vi "Initialize.vi"(8 "error in":errorcluster, 11 "Plugin in":refnum<class "Test Sequencer.lvclass">) -> (0 "error out":errorcluster, 3 "Plugin out":refnum<class "Test Sequencer.lvclass">)   [LabVIEW 2020, in "Test Sequencer.lvlib" / "Test Sequencer.lvclass"]
uses:
  Test Sequencer.lvclass
  C:/Program Files/National Instruments/LabVIEW 2020/vi.lib/FlexLogger/SDK/PluginSDK.lvlibp/PEFClasses/SDK/Plugin/Plugin.lvclass
  <vilib>/FlexLogger/SDK/PluginSDK.lvlibp/PEFClasses/SDK/Processing Element/Timing Parameters.ctl
  <vilib>/FlexLogger/SDK/PluginSDK.lvlibp/PEFClasses/SDK/Processing Element/Timing Method.ctl
  Params.ctl
  Test Sequencer.lvclass/Test Sequencer.ctl
  <vilib>/FlexLogger/SDK/PluginSDK.lvlibp/PEFClasses/SDK/Producer Channel/Producer Channel.lvclass
  C:/Program Files/National Instruments/LabVIEW 2020/vi.lib/FlexLogger/SDK/PluginSDK.lvlibp/PEFClasses/SDK/Channel/Channel.lvclass
  <vilib>/FlexLogger/SDK/PluginSDK.lvlibp/PEFClasses/SDK/Plugin/ParameterAccess/Write Boolean.vi
  <vilib>/FlexLogger/SDK/PluginSDK.lvlibp/PEFClasses/SDK/Plugin/ParameterAccess/Write I32.vi
  <vilib>/FlexLogger/SDK/PluginSDK.lvlibp/PEFClasses/SDK/Plugin/ParameterAccess/Write DBL.vi
  <vilib>/FlexLogger/SDK/PluginSDK.lvlibp/PEFClasses/SDK/Producer Channel/Create Producer Channel.vi
  <vilib>/FlexLogger/SDK/PluginSDK.lvlibp/PEFClasses/SDK/Plugin/Plugin.lvclass
  <vilib>/FlexLogger/SDK/PluginSDK.lvlibp/PEFClasses/SDK/Processing Element/Processing Element.lvclass
  C:/Program Files/National Instruments/LabVIEW 2020/vi.lib/FlexLogger/SDK/PluginSDK.lvlibp/PEFClasses/SDK/Processing Element/Processing Element.lvclass
  \\nirvana\temp/bbuchanan/2020/Test Sequencer.lvclass
  <vilib>/FlexLogger/SDK/PluginSDK.lvlibp
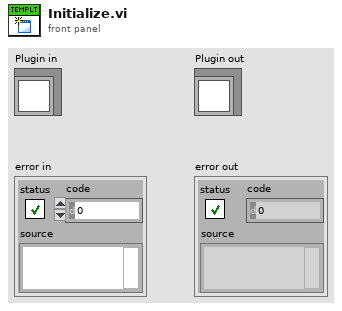
[diagram p1: front panel]
types:
  T1 = typedef "Test Sequencer.lvlib/Test Sequencer.lvclass/Params.ctl" = cluster{"Sequence Durations":dbl[], "Reset on Test Start":bool, "Current Sequence ID":u32, "Total Iterations":u32, "Last Timestamp":timestamp, "Number of Sequence Steps":i32}
  T2 = typedef "PluginSDK.lvlibp/Processing Element.lvclass/Timing Parameters.ctl" = cluster{"Timing Method":T3, "Timing Period (ms)":i32}
  T3 = typedef "PluginSDK.lvlibp/Processing Element.lvclass/Timing Method.ctl" = enum16{"Periodic", "Immediate", "On Data Ready", "Triggered"}
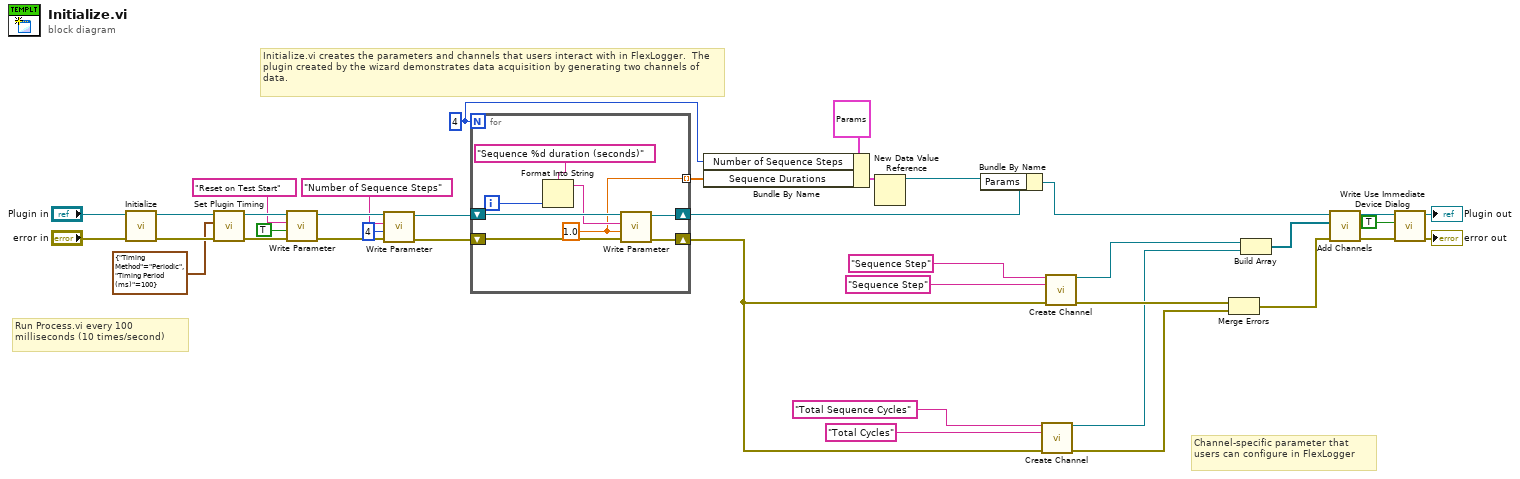
[diagram p0: block diagram]
diagram:
  w15 = 4
  # "Channel-specific parameter that users can configure in FlexLogger"
  # "Run Process.vi every 100 milliseconds (10 times/second)"
  # "Initialize.vi creates the parameters and channels that users interact with in FlexLogger.  The plugin created by the wizard demonstrates data acquisition by generating two channels of data."
  n1 = call-parent "Initialize.vi"("error in (no error)"="error in", "Plugin in"="Plugin in") -> ("error out"=w36:errorcluster, "Plugin out"=w34:refnum<class "Test Sequencer.lvclass">)  [unwired: 8 in]
  n2 = call <vilib>:"Set Plugin Timing.vi"("error in (no error)"=w36, "Timing Parameters"=T2 {"Timing Method"=enum."Periodic", "Timing Period (ms)"=100}, "Plugin in"=w34) -> ("error out"=w30:errorcluster, "Plugin out"=w31:refnum<class "Test Sequencer.lvclass">)  [unwired: 7 in]
  n3 = call-poly <vilib>:"Write Parameter.vi"("error in (no error)"=w30, "Value"=TRUE, "Name"="Reset on Test Start", "Plugin in"=w31) -> ("error out"=w21:errorcluster, "Plugin out"=w20:refnum<class "Test Sequencer.lvclass">)  [unwired: 6 in]
  n4 = call-poly <vilib>:"Write Parameter.vi"("error in (no error)"=w21, "Value"=4, "Name"="Number of Sequence Steps", "Plugin in"=w20) -> ("error out"=w16:errorcluster, "Plugin out"=w17:refnum<class "Test Sequencer.lvclass">)  [unwired: 6 in]
  n5 = for {
    N: w15 -> [_]
    shift-right: [w42] -> w27
    shift-left: w17 -> [w46]
    shift-right: [w41] -> w3
    shift-left: w16 -> [w45]
    tunnel: [w40] -> w25 mode=indexing
    i -> [w39]
    w40 = 1.0 ("Value")
    n6 = Format Into String(format string="Sequence %d duration (seconds)" ("Name"), w39) -> (resulting string=w43:string)  [unwired: 2 in, 1 out]
    n7 = call-poly <vilib>:"Write Parameter.vi"("error in (no error)"=w45, "Value"=w40, "Name"=w43, "Plugin in"=w46) -> ("error out"=w41:errorcluster, "Plugin out"=w42:refnum<class "Test Sequencer.lvclass">)  [unwired: 6 in]
  }
  n8 = Bundle By Name(cluster=T1 {"Sequence Durations"=[], "Reset on Test Start"=TRUE, "Current Sequence ID"=0, "Total Iterations"=0, "Last Timestamp"=timestamp(0 s since 1904-01-01), "Number of Sequence Steps"=0}, "Number of Sequence Steps"=w15, "Sequence Durations"=w25) -> (w24:T1)
  n9 = New Data Value Reference(data value=w24) -> (data value reference=w22:refnum<data-value>)  [unwired: 1 in, 1 out]
  n10 = Bundle By Name(cluster=w27, "Params"=w22) -> (w23:refnum<class "Test Sequencer.lvclass">)
  n11 = call-poly <vilib>:"Create Channel.vi"("Unique Channel Identifier"="Total Sequence Cycles" ("format string"), "Default Channel Name"="Total Cycles" ("format string"), "error in (no error)"=w3) -> ("Producer Channel"=w1:refnum<class "Producer Channel.lvclass">, "error out"=w2:errorcluster)  [unwired: 11 in]
  n12 = call-poly <vilib>:"Create Channel.vi"("Unique Channel Identifier"="Sequence Step" ("format string"), "Default Channel Name"="Sequence Step" ("format string"), "error in (no error)"=w3) -> ("Producer Channel"=w6:refnum<class "Producer Channel.lvclass">, "error out"=w7:errorcluster)  [unwired: 11 in]
  n13 = Merge Errors(w7, w2) -> (w32:errorcluster)
  n14 = Build Array(w6, w1) -> (w33:refnum<class "Producer Channel.lvclass">[])
  n15 = call <vilib>:"Add Channels.vi"("error in (no error)"=w32, "Channels"=w33, "Plugin in"=w23) -> ("error out"=w13:errorcluster, "Plugin out"=w14:refnum<class "Test Sequencer.lvclass">)  [unwired: 7 in]
  n16 = call <vilib>:"Write Use Immediate Device Dialog.vi"("error in (no error)"=w13, "Use Immediate Device Dialog?"=TRUE, "Plugin in"=w14) -> ("error out"=→"error out":errorcluster, "Plugin out"=→"Plugin out":refnum<class "Test Sequencer.lvclass">)  [unwired: 7 in]
